vi "test_isRunningValidation.vi"(11 "Test Case In":refnum<class "TaskControllerTests.lvclass">) -> (0 "error out":errorcluster, 3 "Test Case Out":refnum<class "TaskControllerTests.lvclass">)   [LabVIEW 2023, in "TaskControllerTests.lvclass"]
uses:
  TaskControllerTests.lvclass
  TaskControllerTests.lvclass/TaskControllerTests.ctl
  TaskMock/TaskMock.lvclass
  <vilib>/Astemes/LUnit/Test Case.lvclass
  source/TaskController/TaskController.lvclass
  C:/projects/TLC_Daemon/tests/TaskMock/TaskMock.lvclass
  C:/projects/TLC_Daemon/source/ITask/ITask.lvclass
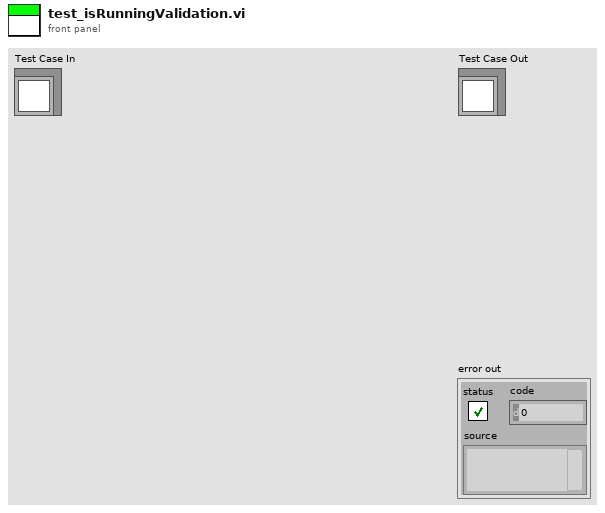
[diagram p1: front panel]
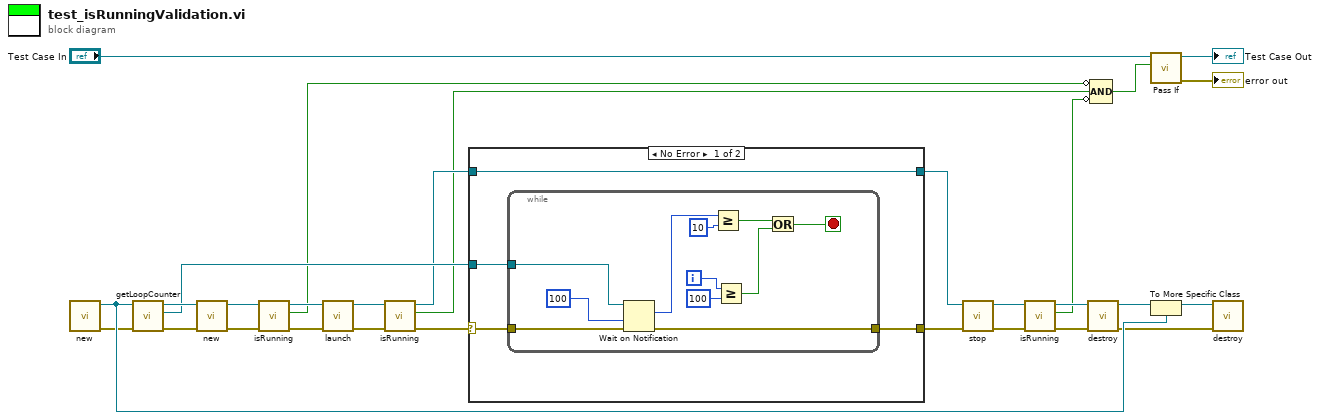
[diagram p0: block diagram]
diagram:
  n1 = call "new.vi"() -> ("error out"=w17:errorcluster, "TaskMock out"=w21:refnum<class "TaskMock.lvclass">)  [unwired: 10 in]
  n2 = call "getLoopCounter.vi"("error in (no error)"=w17, "TaskMock in"=w21) -> ("error out"=w16:errorcluster, "loopCounter"=w24:refnum<notifier>, "TaskMock out"=w25:refnum<class "TaskMock.lvclass">)  [unwired: 7 in]
  n3 = call "new.vi"("error in (no error)"=w16, "task"=w25) -> ("error out"=w26:errorcluster, "TaskController out"=w14:refnum<class "TaskController.lvclass">)  [unwired: 8 in]
  n4 = call "isRunning.vi"("error in (no error)"=w26, "TaskController in"=w14) -> ("error out"=w15:errorcluster, "isRunning"=w4:bool, "TaskController out"=w13:refnum<class "TaskController.lvclass">)  [unwired: 7 in]
  n5 = call "launch.vi"("error in (no error)"=w15, "TaskController in"=w13) -> ("error out"=w12:errorcluster, "TaskController out"=w10:refnum<class "TaskController.lvclass">)  [unwired: 8 in]
  n6 = call "isRunning.vi"("error in (no error)"=w12, "TaskController in"=w10) -> ("error out"=w11:errorcluster, "isRunning"=w3:bool, "TaskController out"=w9:refnum<class "TaskController.lvclass">)  [unwired: 7 in]
  n7 = case shown="No Error" w11 {
    selector: w11 -> [w33 _]
    tunnel: w9 -> [w31 w45]
    tunnel: w24 -> [w32 _]
    tunnel: [w31 w45] -> w23
    tunnel: [w30 _] -> w22
    frame No Error {
      n8 = while {
        tunnel: w33 -> [w35]
        tunnel: w32 -> [w44]
        tunnel: [w34] -> w30
        i -> [w40]
        stop <- w37 stop-if-true
        n9 = Wait on Notification(notifier=w44, timeout in ms (-1)=100, error in (no error)=w35) -> (notification=w42:i32, error out=w34:errorcluster)  [unwired: 1 in, 2 out]
        n10 = Greater Or Equal?(x=w42, y=10) -> (x >= y?=w38:bool)
        n11 = Greater Or Equal?(x=w40, y=100) -> (x >= y?=w36:bool)
        n12 = Or(x=w38, y=w36) -> (x .or. y?=w37:bool)
      }
    }
    frame Error {
    }
  }
  n13 = call "stop.vi"("error in (no error)"=w22, "TaskController in"=w23) -> ("error out"=w8:errorcluster, "TaskController out"=w6:refnum<class "TaskController.lvclass">)  [unwired: 8 in]
  n14 = call "isRunning.vi"("error in (no error)"=w8, "TaskController in"=w6) -> ("error out"=w7:errorcluster, "isRunning"=w2:bool, "TaskController out"=w5:refnum<class "TaskController.lvclass">)  [unwired: 7 in]
  n15 = call "destroy.vi"("error in (no error)"=w7, "TaskController in"=w5) -> ("error out"=w20:errorcluster, "task"=w19:refnum<class "ITask.lvclass">)  [unwired: 8 in]
  n16 = Compound Arithmetic op=AND(invert w4, w3, invert w2) -> (w1:bool)
  n17 = call <vilib>:"Pass If.vi"("Pass?"=w1, "LUnit Test Case In"="Test Case In") -> ("error out"=→"error out":errorcluster, "LUnit Test Case Out"=→"Test Case Out":refnum<class "TaskControllerTests.lvclass">)  [unwired: 8 in]
  n18 = To More Specific Class(target class=w21, reference=w19) -> (specific class reference=w18:refnum<class "TaskMock.lvclass">)  [unwired: 1 in, 1 out]
  n19 = call "destroy.vi"("error in (no error)"=w20, "TaskMock in"=w18) -> ()  [unwired: 9 in, 1 out]
